vi "Set Operating Mode.vi"(7 "Operating mode":T1=enum."Single Stepping", 8 "error in (no error)":errorcluster, 11 "CD Ref in":T2 format="%.0x") -> (0 "error out":errorcluster, 3 "Item Ref out":T2 format="%.0x")   [LabVIEW 2019, in "TimingDRV System Explorer.lvlib"]
uses:
  TimingDRV System Explorer.lvlib
  <vilib>/NI VeriStand/Custom Device API/Custom Device Item Ref.ctl
  TypeDefs/Operating Mode Types.ctl
  Engine/Parent Classes/Process/Process.lvclass
  Engine/Processes/Single Stepped TS/STS Process.lvclass
  C:/Users/XEnderMD/Desktop/CD Project Tools/Source/Engine/Parent Classes/Process/Process.lvclass
  Engine/Processes/TCP Process/TCP Process.lvclass
  Engine/Processes/Free Running TS/FRTS Process.lvclass
  <vilib>/NI VeriStand/Custom Device API/Set Item Property (String).vi
  <vilib>/NI VeriStand/Custom Device API/Set Item Property (I32).vi
  <vilib>/NI VeriStand/Custom Device API/Custom Device API.lvlib
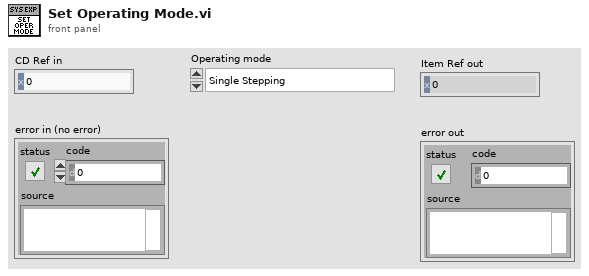
[diagram p1: front panel]
types:
  T1 = typedef "TimingDRV System Explorer.lvlib/Operating Mode Types.ctl" = enum16{"Free Running", "Single Stepping"}
  T2 = typedef "Custom Device API.lvlib/Custom Device Item Ref.ctl" = u64
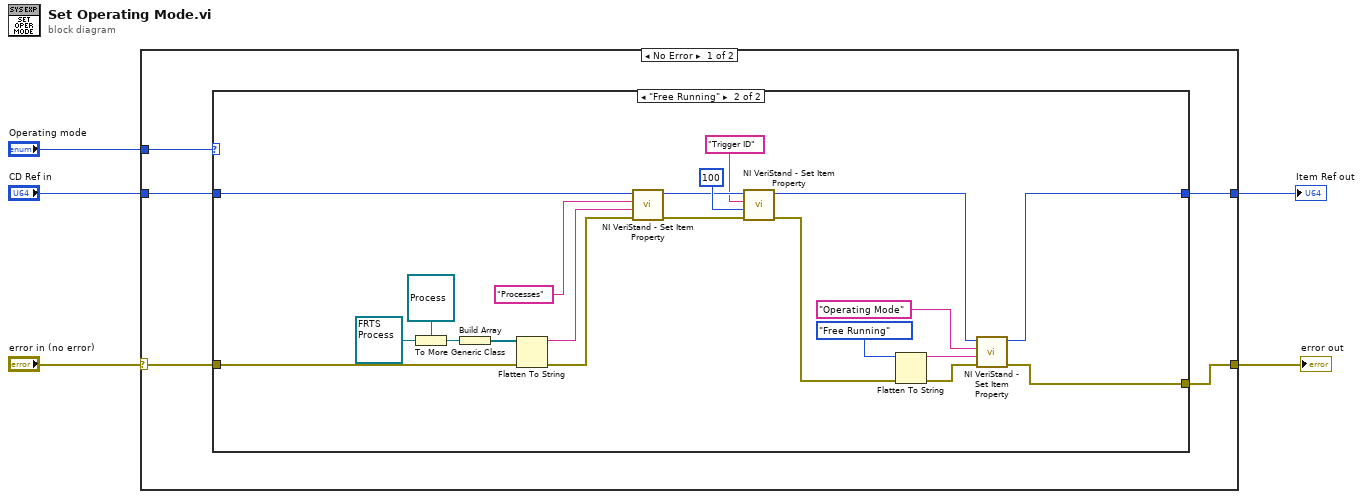
[diagram p0: block diagram]
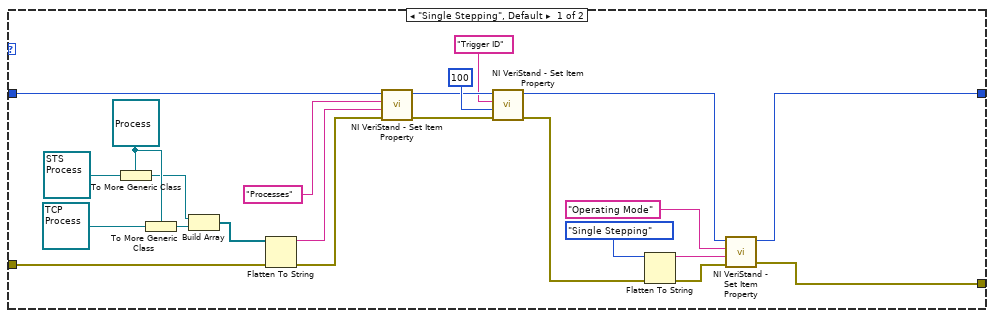
[diagram p2: hidden frame]
diagram:
  n1 = case shown="No Error" "error in (no error)" {
    selector: "error in (no error)" -> [w7 w55]
    tunnel: [w10 w56] -> w5
    tunnel: [w9 w55] -> w4
    tunnel: "CD Ref in" -> [w8 w56]
    tunnel: "Operating mode" -> [w6 _]
    frame No Error {
      n2 = case shown="\"Free Running\"" w6 {
        tunnel: [w33 w54] -> w10
        tunnel: [w11 w47] -> w9
        tunnel: w8 -> [w20 w44]
        tunnel: w7 -> [w12 w34]
        frame "Single Stepping", Default {
          w25 = refnum<class "Process.lvclass"> refnum ("TelemetryAsync Engine.lvlib:Process.lvclass")
          n3 = To More Generic Class(target class=w25, reference=refnum<class "STS Process.lvclass"> refnum ("TimingDRV Engine.lvlib:STS Process.lvclass")) -> (generic class reference=w22:refnum<class "Process.lvclass">)
          n4 = To More Generic Class(target class=w25, reference=refnum<class "TCP Process.lvclass"> refnum ("TimingDRV Engine.lvlib:TCP Process.lvclass")) -> (generic class reference=w26:refnum<class "Process.lvclass">)
          n5 = Build Array(w22, w26) -> (w23:refnum<class "Process.lvclass">[])
          n6 = Flatten To String(anything=w23, error in (no error)=w12) -> (data string=w14:string, error out=w15:errorcluster)  [unwired: 2 in, 1 out]
          n7 = call-poly <vilib>:"NI VeriStand - Set Item Property.vi"("error in (no error)"=w15, "Value"=w14, "Property Name"="Processes", "Item Ref in"=w20) -> ("error out"=w18:errorcluster, "Item Ref out"=w17:T2)  [unwired: 5 in, 1 out]
          n8 = call-poly <vilib>:"NI VeriStand - Set Item Property.vi"("error in (no error)"=w18, "Value"=100, "Property Name"="Trigger ID", "Item Ref in"=w17) -> ("error out"=w29:errorcluster, "Item Ref out"=w27:T2)  [unwired: 5 in, 1 out]
          n9 = Flatten To String(anything=Operating_Mode_Types."Single Stepping" ("Operating mode"), error in (no error)=w29) -> (data string=w31:string, error out=w30:errorcluster)  [unwired: 2 in, 1 out]
          n10 = call-poly <vilib>:"NI VeriStand - Set Item Property.vi"("error in (no error)"=w30, "Value"=w31, "Property Name"="Operating Mode", "Item Ref in"=w27) -> ("error out"=w11:errorcluster, "Item Ref out"=w33:T2)  [unwired: 5 in, 1 out]
        }
        frame "Free Running" {
          n11 = To More Generic Class(target class=refnum<class "Process.lvclass"> refnum ("TelemetryAsync Engine.lvlib:Process.lvclass"), reference=refnum<class "FRTS Process.lvclass"> refnum ("TimingDRV Engine.lvlib:FRTS Process.lvclass")) -> (generic class reference=w45:refnum<class "Process.lvclass">)
          n12 = Build Array(w45) -> (w46:refnum<class "Process.lvclass">[])
          n13 = Flatten To String(anything=w46, error in (no error)=w34) -> (data string=w38:string, error out=w39:errorcluster)  [unwired: 2 in, 1 out]
          n14 = call-poly <vilib>:"NI VeriStand - Set Item Property.vi"("error in (no error)"=w39, "Value"=w38, "Property Name"="Processes", "Item Ref in"=w44) -> ("error out"=w42:errorcluster, "Item Ref out"=w41:T2)  [unwired: 5 in, 1 out]
          n15 = call-poly <vilib>:"NI VeriStand - Set Item Property.vi"("error in (no error)"=w42, "Value"=100, "Property Name"="Trigger ID", "Item Ref in"=w41) -> ("error out"=w50:errorcluster, "Item Ref out"=w48:T2)  [unwired: 5 in, 1 out]
          n16 = Flatten To String(anything=Operating_Mode_Types."Free Running" ("Operating mode"), error in (no error)=w50) -> (data string=w52:string, error out=w51:errorcluster)  [unwired: 2 in, 1 out]
          n17 = call-poly <vilib>:"NI VeriStand - Set Item Property.vi"("error in (no error)"=w51, "Value"=w52, "Property Name"="Operating Mode", "Item Ref in"=w48) -> ("error out"=w47:errorcluster, "Item Ref out"=w54:T2)  [unwired: 5 in, 1 out]
        }
      }
    }
    frame Error {
    }
  }
  "Item Ref out" <- w5
  "error out" <- w4
